vi "tm420_sequence.vi"() -> ()   [LabVIEW 2023, in "HamamatsuCam.lvlib" / "HamamatsuCam.lvclass"]
uses:
  HamamatsuCam/HamamatsuCam/HamamatsuCam.lvclass
panel:
  out "Waveform Graph":u16[](graph)
  out "Timestamp":dbl
  out "DCAM Version":string
  out "Library Version":string
  out "Image":u16[][](graph)
  out "Frames Per Second":dbl
  in  "Quit":bool
  out "Error Out":errorcluster {"code" format="%.0x"}
  # "This is just a simple example\nof how to capture and display\nlive data."
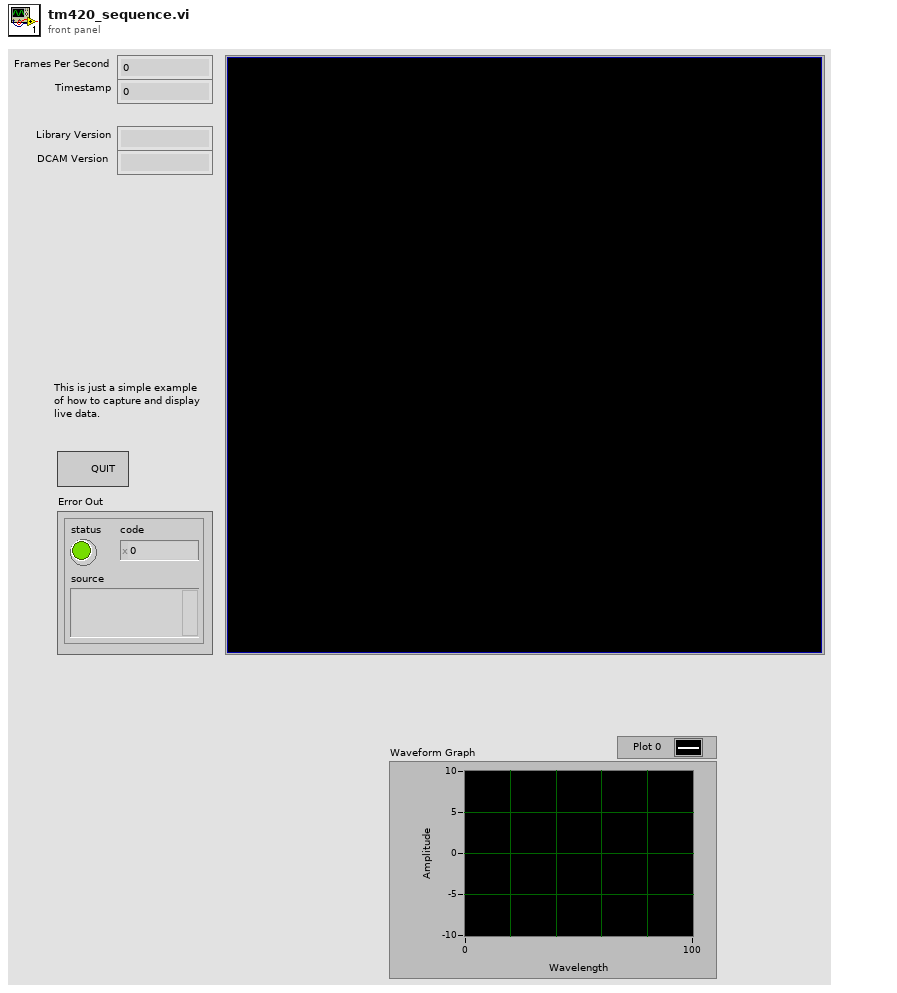
[diagram p1: front panel]
types:
  T1 = cluster{"Capture Library":string, "DCAM-API":string}
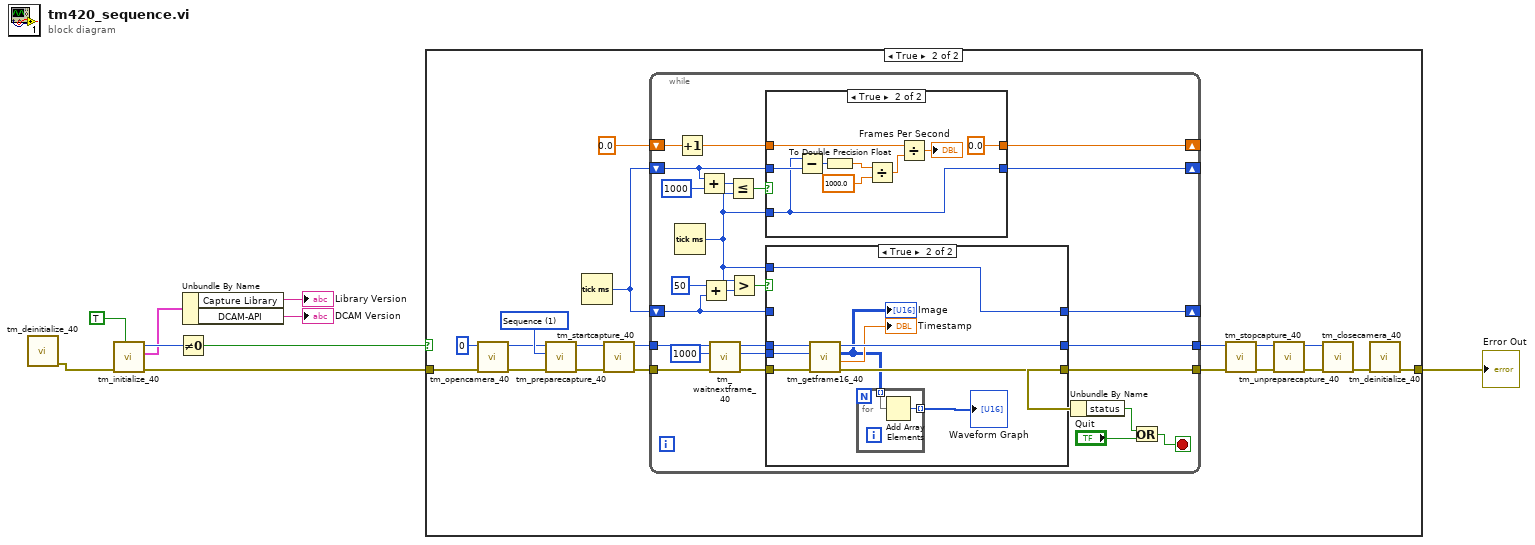
[diagram p0: block diagram]
diagram:
  n1 = call "tm_deinitialize_40.vi"() -> ("error out"=w2:errorcluster)  [unwired: 11 in]
  n2 = call "tm_initialize_40.vi"("HVCC Log (F)"=TRUE, "error in (no error)"=w2) -> ("error out"=w7:errorcluster, "Version Info"=w6:T1, "Number Of Cameras"=w8:u32)  [unwired: 6 in, 1 out]
  n3 = Not Equal To 0?(x=w8) -> (x != 0?=w9:bool)
  n4 = Unbundle By Name(w6) -> ("Capture Library"=→"Library Version":string, "DCAM-API"=→"DCAM Version":string)
  n5 = case shown="True" w9 {
    tunnel: w7 -> [w10 w29]
    tunnel: [w10 w11] -> w3
    frame False {
    }
    frame True {
      w19 = 1 items=["Snap", "Sequence"] ("Capture mode")
      n6 = call "tm_opencamera_40.vi"("error in (no error)"=w29, "Camera Index"=u32 0) -> ("error out"=w13:errorcluster, "Handle out"=w14:u32)  [unwired: 7 in, 1 out]
      n7 = call "tm_preparecapture_40.vi"("error in (no error)"=w13, "Capture mode"=w19, "Handle in"=w14) -> ("error out"=w17:errorcluster, "Handle out"=w18:u32)  [unwired: 5 in, 2 out]
      n8 = Tick Count (ms)() -> (millisecond timer value=w15:u32)
      n9 = call "tm_startcapture_40.vi"("error in (no error)"=w17, "Handle in"=w18) -> ("error out"=w20:errorcluster, "Handle out"=w21:u32)  [unwired: 8 in]
      n10 = while {
        tunnel: [w33] -> w24
        tunnel: [w34] -> w25
        tunnel: w21 -> [w51]
        tunnel: w20 -> [w52]
        shift-right: [w49] -> _
        shift-left: w15 -> [w46]
        shift-right: [w50] -> _
        shift-left: 0.0 -> [w43]
        shift-right: [w32] -> _
        shift-left: w15 -> [w35]
        stop <- w31 stop-if-true
        n11 = Tick Count (ms)() -> (millisecond timer value=w36:u32)
        n12 = Increment(x=w43) -> (x+1=w44:dbl)
        n13 = Add(x=w46, y=u32 1000) -> (x+y=w48:u32)
        n14 = Add(x=u32 50, y=w35) -> (x+y=w38:u32)
        n15 = call "tm_waitnextframe_40.vi"("error in (no error)"=w52, "Timeout"=1000, "Handle in"=w51) -> ("error out"=w41:errorcluster, "Frame Index"=w40:i32, "Handle out"=w42:u32)  [unwired: 5 in, 1 out]
        n16 = Less Or Equal?(x=w48, y=w36) -> (x <= y?=w45:bool)
        n17 = Greater?(x=w36, y=w38) -> (0:w37:bool)
        n18 = case shown="True" w45 {
          tunnel: w46 -> [w70 w73]
          tunnel: [w70 w71] -> w49
          tunnel: w44 -> [w69 w77]
          tunnel: w36 -> [_ w71]
          tunnel: [w69 0.0] -> w50
          frame False {
          }
          frame True {
            n19 = Subtract(x=w71, y=w73) -> (x-y=w72:u32)
            n20 = To Double Precision Float(number=w72) -> (double precision float=w79:dbl)
            n21 = Divide(x=w79, y=1000.0) -> (x/y=w76:dbl)
            n22 = Divide(x=w77, y=w76) -> (x/y=→"Frames Per Second":dbl)
          }
        }
        n23 = case shown="True" w37 {
          tunnel: w42 -> [w57 w66]
          tunnel: w41 -> [w56 w65]
          tunnel: w40 -> [_ w60]
          tunnel: w35 -> [w55 _]
          tunnel: w36 -> [_ w64]
          tunnel: [w57 w62] -> w33
          tunnel: [w56 w63] -> w34
          tunnel: [w55 w64] -> w32
          frame False {
          }
          frame True {
            n24 = call "tm_getframe16_40.vi"("error in (no error)"=w65, "Frame Index"=w60, "Handle in"=w66) -> ("error out"=w63:errorcluster, "Timestamp"=→"Timestamp":dbl, "Data"=w59:u16[][], "Handle out"=w62:u32)  [unwired: 5 in]
            "Image" <- w59
            n25 = for {
              tunnel: [w68] -> w58 mode=indexing
              tunnel: w59 -> [w67] mode=indexing
              n26 = Add Array Elements(numeric array=w67) -> (sum=w68:u16)
            }
            "Waveform Graph" <- w58
          }
        }
        n27 = Unbundle By Name(w34) -> ("status"=w54:bool)
        n28 = Or(x=w54, y="Quit") -> (x .or. y?=w31:bool)
      }
      n29 = call "tm_stopcapture_40.vi"("error in (no error)"=w25, "Handle in"=w24) -> ("error out"=w22:errorcluster, "Handle out"=w23:u32)  [unwired: 8 in]
      n30 = call "tm_unpreparecapture_40.vi"("error in (no error)"=w22, "Handle in"=w23) -> ("error out"=w27:errorcluster, "Handle out"=w26:u32)  [unwired: 8 in]
      n31 = call "tm_closecamera_40.vi"("error in (no error)"=w27, "Handle in"=w26) -> ("error out"=w12:errorcluster)  [unwired: 9 in]
      n32 = call "tm_deinitialize_40.vi"("error in (no error)"=w12) -> ("error out"=w11:errorcluster)  [unwired: 10 in]
    }
  }
  "Error Out" <- w3
